vi "nipkg-setPackageVersion.vi"(8 "error in (no error)":errorcluster, 10 "Package Version":string, 11 "Project refs":T1={"LabVIEW Project Path"=path "C:/Users/admin/Desktop/Source/Waveform-Processing-Custom-Device.lvproj", "Project refnum"=refnum, "Build spec refnum"=refnum}) -> (0 "error out":errorcluster, 3 "Project refs out":T1={"LabVIEW Project Path"=path "C:/Users/admin/Desktop/Source/Waveform-Processing-Custom-Device.lvproj", "Project refnum"=refnum, "Build spec refnum"=refnum})   [LabVIEW 2014, in "nipkg-build-system.lvlib"]
uses:
  nipkg-build-system.lvlib
  lv-build-system/lv-build-library.lvlib
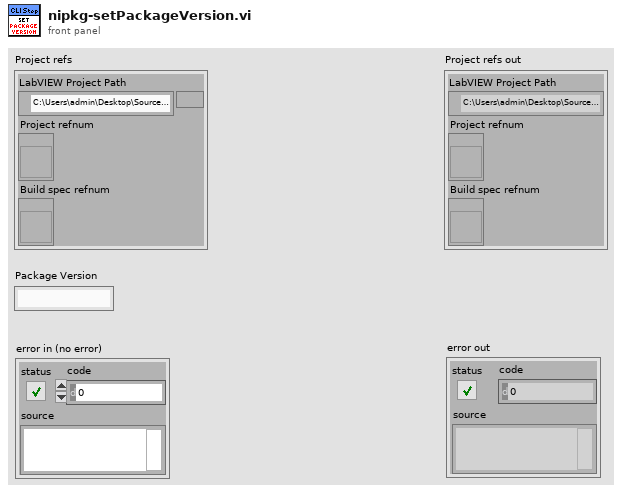
[diagram p1: front panel]
types:
  T1 = cluster{"LabVIEW Project Path":path, "Project refnum":refnum<vi>, "Build spec refnum":refnum<vi>}
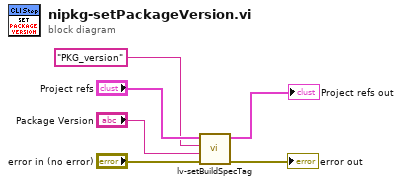
[diagram p0: block diagram]
diagram:
  n1 = call "lv-setBuildSpecTag.vi"("error in (no error)"="error in (no error)", "Tag value"="Package Version", "Tag name"="PKG_version", "Project refs"="Project refs") -> ("error out"=→"error out":errorcluster, "Project refs out"=→"Project refs out":T1)  [unwired: 6 in]
